vi "Run_Core.vi"(0 "Bitwise Operations in":refnum<class "Bitwise Functions.lvclass">, 11 "error in (no error)":errorcluster) -> (4 "Bitwise Operations out":refnum<class "Bitwise Functions.lvclass">, 6 "Return":variant, 15 "error out":errorcluster)   [LabVIEW 2019, in "Bitwise Functions.lvclass"]
uses:
  Bitwise Functions.lvclass
  Bitwise Functions.lvclass/Bitwise Functions.ctl
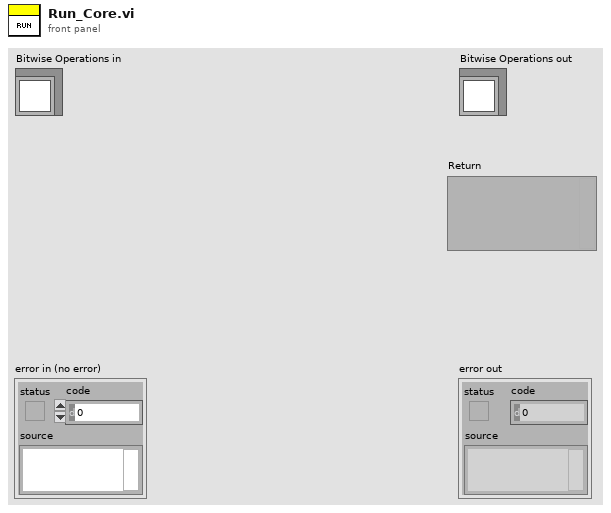
[diagram p1: front panel]
types:
  T1 = typedef "Bitwise Functions.lvclass/Function List.ctl" = enum16{"Bitwise And", "Bitwise Or", "Bitwise ExOR", "One's Compliment", "Shift Left", "Shift Right"}
  T2 = typedef "Datatype.ctl" = enum16{"Null", "Numeric", "String", "Bool", "Numeric 1D", "String 1D", "Bool 1D", "Numeric 2D", "String 2D", "Bool 2D", "Variant"}
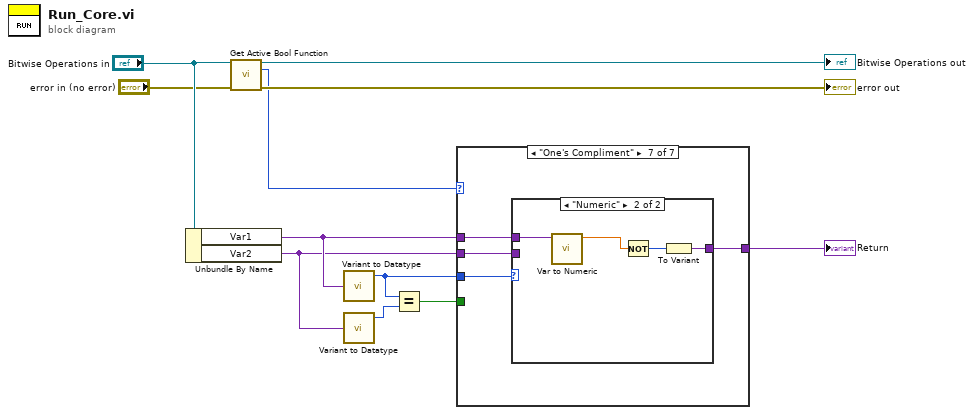
[diagram p0: block diagram]
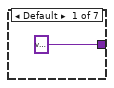
[diagram p2: hidden frame]
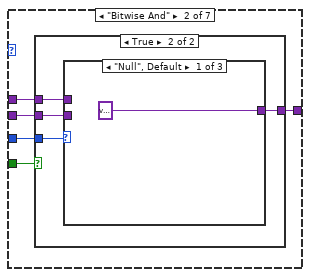
[diagram p3: hidden frame]
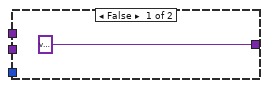
[diagram p4: hidden frame]
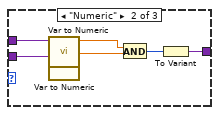
[diagram p5: hidden frame]
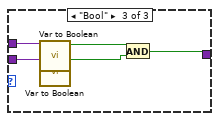
[diagram p6: hidden frame]
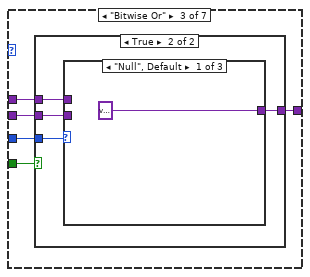
[diagram p7: hidden frame]
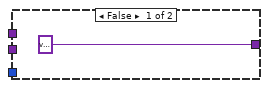
[diagram p8: hidden frame]
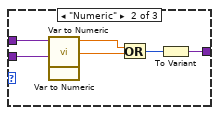
[diagram p9: hidden frame]
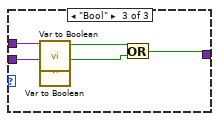
[diagram p10: hidden frame]
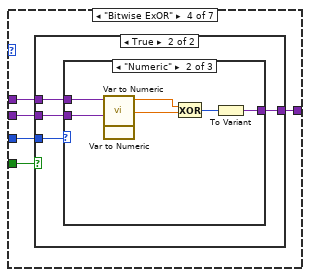
[diagram p11: hidden frame]
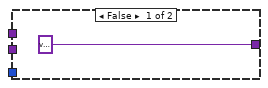
[diagram p12: hidden frame]
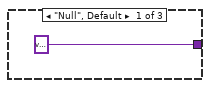
[diagram p13: hidden frame]
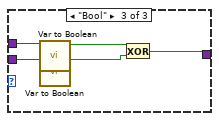
[diagram p14: hidden frame]
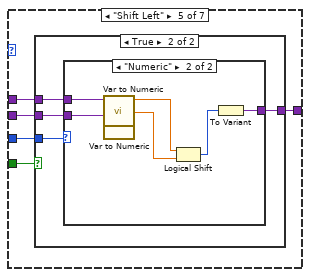
[diagram p15: hidden frame]
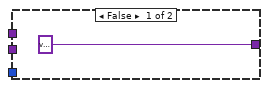
[diagram p16: hidden frame]
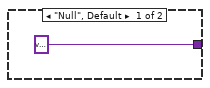
[diagram p17: hidden frame]
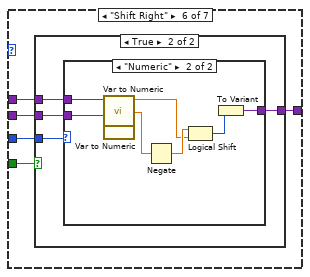
[diagram p18: hidden frame]
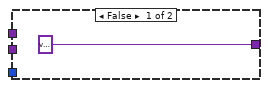
[diagram p19: hidden frame]
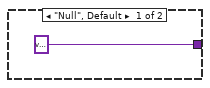
[diagram p20: hidden frame]
diagram:
  n1 = Unbundle By Name("Bitwise Operations in") -> ("Var1"=w5:variant, "Var2"=w4:variant)
  n2 = call "Get Active Bool Function.vi"("Bitwise Functions in"="Bitwise Operations in", "error in (no error)"="error in (no error)") -> ("Bitwise Functions out"=→"Bitwise Operations out":refnum<class "Bitwise Functions.lvclass">, "Function"=w6:T1, "error out"=→"error out":errorcluster)  [unwired: 11 in]
  n3 = call "Variant to Datatype.vi"("Variant"=w5) -> ("Datatype"=w1:T2)  [unwired: 2 in, 2 out]
  n4 = call "Variant to Datatype.vi"("Variant"=w4) -> ("Datatype"=w3:T2)  [unwired: 2 in, 2 out]
  n5 = Equal?(x=w1, y=w3) -> (x = y?=w2:bool)
  n6 = case shown="\"One's Compliment\"" w6 {
    tunnel: w5 -> [_ w15 w37 w59 w81 w98 w116]
    tunnel: w4 -> [_ w14 w36 w58 w80 w97 w115]
    tunnel: [variant ("Variant") w17 w39 w61 w83 w100 w117] -> w11
    tunnel: w2 -> [_ w16 w38 w60 w82 w99 _]
    tunnel: w1 -> [_ w13 w35 w57 w79 w96 w114]
    frame Default {
    }
    frame "Bitwise And" {
      n7 = case shown="True" w16 {
        tunnel: [variant ("Variant") w22] -> w17
        tunnel: w15 -> [_ w20]
        tunnel: w14 -> [_ w19]
        tunnel: w13 -> [_ w21]
        frame False {
        }
        frame True {
          n8 = case shown="\"Null\", Default" w21 {
            tunnel: [variant ("Variant") w28 w30] -> w22
            tunnel: w20 -> [_ w27 w34]
            tunnel: w19 -> [_ w26 w33]
            frame "Null", Default {
            }
            frame "Numeric" {
              n9 = call "Var to Numeric.vi"("Variant"=w27) -> ("Numeric"=w24:dbl)  [unwired: 10 in]
              n10 = call "Var to Numeric.vi"("Variant"=w26) -> ("Numeric"=w25:dbl)  [unwired: 10 in]
              n11 = And(x=w24, y=w25) -> (x .and. y?=w29:i32)
              n12 = To Variant(anything=w29) -> (Variant=w28:variant)
            }
            frame "Bool" {
              n13 = call "Var to Boolean.vi"("Variant"=w34) -> ("Boolean"=w32:bool)  [unwired: 10 in]
              n14 = call "Var to Boolean.vi"("Variant"=w33) -> ("Boolean"=w31:bool)  [unwired: 10 in]
              n15 = And(x=w32, y=w31) -> (x .and. y?=w30:bool)
            }
          }
        }
      }
    }
    frame "Bitwise Or" {
      n16 = case shown="True" w38 {
        tunnel: [variant ("Variant") w44] -> w39
        tunnel: w37 -> [_ w42]
        tunnel: w36 -> [_ w41]
        tunnel: w35 -> [_ w43]
        frame False {
        }
        frame True {
          n17 = case shown="\"Null\", Default" w43 {
            tunnel: [variant ("Variant") w50 w52] -> w44
            tunnel: w42 -> [_ w49 w56]
            tunnel: w41 -> [_ w48 w55]
            frame "Null", Default {
            }
            frame "Numeric" {
              n18 = call "Var to Numeric.vi"("Variant"=w49) -> ("Numeric"=w46:dbl)  [unwired: 10 in]
              n19 = call "Var to Numeric.vi"("Variant"=w48) -> ("Numeric"=w47:dbl)  [unwired: 10 in]
              n20 = Or(x=w46, y=w47) -> (x .or. y?=w51:i32)
              n21 = To Variant(anything=w51) -> (Variant=w50:variant)
            }
            frame "Bool" {
              n22 = call "Var to Boolean.vi"("Variant"=w56) -> ("Boolean"=w54:bool)  [unwired: 10 in]
              n23 = call "Var to Boolean.vi"("Variant"=w55) -> ("Boolean"=w53:bool)  [unwired: 10 in]
              n24 = Or(x=w54, y=w53) -> (x .or. y?=w52:bool)
            }
          }
        }
      }
    }
    frame "Bitwise ExOR" {
      n25 = case shown="True" w60 {
        tunnel: [variant ("Variant") w66] -> w61
        tunnel: w59 -> [_ w64]
        tunnel: w58 -> [_ w63]
        tunnel: w57 -> [_ w65]
        frame False {
        }
        frame True {
          n26 = case shown="\"Numeric\"" w65 {
            tunnel: [variant ("Variant") w72 w74] -> w66
            tunnel: w64 -> [_ w71 w78]
            tunnel: w63 -> [_ w70 w77]
            frame "Null", Default {
            }
            frame "Numeric" {
              n27 = call "Var to Numeric.vi"("Variant"=w71) -> ("Numeric"=w68:dbl)  [unwired: 10 in]
              n28 = call "Var to Numeric.vi"("Variant"=w70) -> ("Numeric"=w69:dbl)  [unwired: 10 in]
              n29 = Exclusive Or(1:w69, 2:w68) -> (0:w73:i32)
              n30 = To Variant(anything=w73) -> (Variant=w72:variant)
            }
            frame "Bool" {
              n31 = call "Var to Boolean.vi"("Variant"=w78) -> ("Boolean"=w76:bool)  [unwired: 10 in]
              n32 = call "Var to Boolean.vi"("Variant"=w77) -> ("Boolean"=w75:bool)  [unwired: 10 in]
              n33 = Exclusive Or(1:w75, 2:w76) -> (0:w74:bool)
            }
          }
        }
      }
    }
    frame "Shift Left" {
      n34 = case shown="True" w82 {
        tunnel: [variant ("Variant") w88] -> w83
        tunnel: w81 -> [_ w86]
        tunnel: w80 -> [_ w85]
        tunnel: w79 -> [_ w87]
        frame False {
        }
        frame True {
          n35 = case shown="\"Numeric\"" w87 {
            tunnel: [variant ("Variant") w95] -> w88
            tunnel: w86 -> [_ w94]
            tunnel: w85 -> [_ w93]
            frame "Null", Default {
            }
            frame "Numeric" {
              n36 = call "Var to Numeric.vi"("Variant"=w94) -> ("Numeric"=w92:dbl)  [unwired: 10 in]
              n37 = call "Var to Numeric.vi"("Variant"=w93) -> ("Numeric"=w91:dbl)  [unwired: 10 in]
              n38 = Logical Shift(y=w92, x=w91) -> (x << y=w90:u32)
              n39 = To Variant(anything=w90) -> (Variant=w95:variant)
            }
          }
        }
      }
    }
    frame "Shift Right" {
      n40 = case shown="True" w99 {
        tunnel: [variant ("Variant") w105] -> w100
        tunnel: w98 -> [_ w103]
        tunnel: w97 -> [_ w102]
        tunnel: w96 -> [_ w104]
        frame False {
        }
        frame True {
          n41 = case shown="\"Numeric\"" w104 {
            tunnel: [variant ("Variant") w113] -> w105
            tunnel: w103 -> [_ w112]
            tunnel: w102 -> [_ w111]
            frame "Null", Default {
            }
            frame "Numeric" {
              n42 = call "Var to Numeric.vi"("Variant"=w112) -> ("Numeric"=w109:dbl)  [unwired: 10 in]
              n43 = call "Var to Numeric.vi"("Variant"=w111) -> ("Numeric"=w108:dbl)  [unwired: 10 in]
              n44 = Negate(x=w108) -> (-x=w110:dbl)
              n45 = Logical Shift(y=w110, x=w109) -> (x << y=w107:u32)
              n46 = To Variant(anything=w107) -> (Variant=w113:variant)
            }
          }
        }
      }
    }
    frame "One's Compliment" {
      n47 = case shown="\"Numeric\"" w114 {
        tunnel: [variant ("Variant") w121] -> w117
        tunnel: w116 -> [_ w120]
        tunnel: w115 -> [_ _]
        frame "Null", Default {
        }
        frame "Numeric" {
          n48 = call "Var to Numeric.vi"("Variant"=w120) -> ("Numeric"=w119:dbl)  [unwired: 10 in]
          n49 = Not(x=w119) -> (.not. x?=w122:u32)
          n50 = To Variant(anything=w122) -> (Variant=w121:variant)
        }
      }
    }
  }
  "Return" <- w11
